vi "mqttCmdConnectClassRead.vi"(0 "mqttConnect in":refnum<class "mqttCmdConnect.lvclass">, 11 "error in (no error)":errorcluster) -> (4 "mqttConnect out":refnum<class "mqttCmdConnect.lvclass">, 6 "mqtt.lvclass":refnum<class "mqtt.lvclass">, 15 "error out":errorcluster)   [LabVIEW 2022 SP3, in "mqttCmdConnect.lvclass"]
uses:
  mqttCmdConnect.lvclass
  mqtt.lvclass
  mqttCmdConnect.lvclass/mqttCmdConnect.ctl
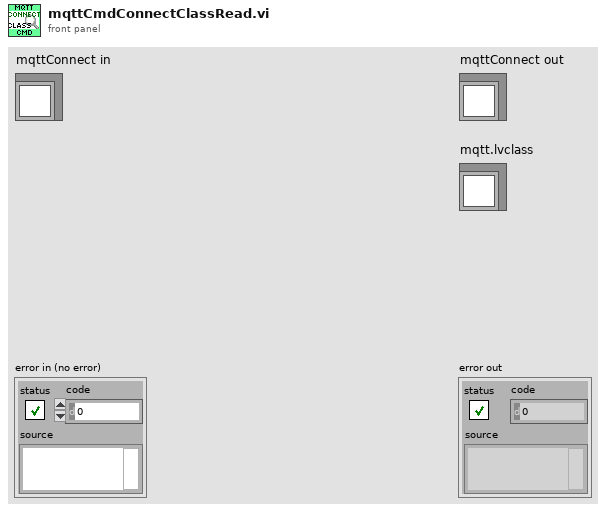
[diagram p1: front panel]
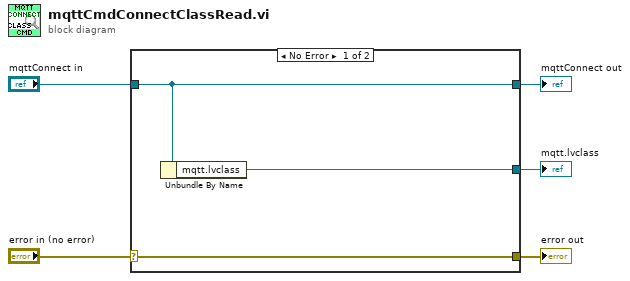
[diagram p0: block diagram]
diagram:
  n1 = case shown="No Error" "error in (no error)" {
    selector: "error in (no error)" -> [w8 w9]
    tunnel: [w8 w9] -> w4
    tunnel: [w7 w10] -> w2
    tunnel: "mqttConnect in" -> [w7 w10]
    tunnel: [w6 _] -> w1
    frame No Error {
      n2 = Unbundle By Name(w7) -> ("mqtt.lvclass"=w6:refnum<class "mqtt.lvclass">)
    }
    frame Error {
    }
  }
  "error out" <- w4
  "mqttConnect out" <- w2
  "mqtt.lvclass" <- w1
